vi "Main.vi"() -> ()   [LabVIEW 2025]
uses:
  TypeDef_AuxPlotValues.ctl
  TypeDef_AuxDataToDisplay.ctl
  TypeDef_Modes.ctl
  TypeDef_BBBJSON_commands.ctl
  TypeDef_Network.ctl
  <vilib>/Analysis/1siggen.llb/Ramp Pattern by Samples.vi
  <vilib>/Analysis/NI_AALBase.lvlib
panel:
  out "Gly Conc (ppb)":dbl
  out "NO2 Conc (ppb)":dbl
  out "Laptop loop time":dbl
  out "Laptop Time":timestamp
  out "Aux data to display":T1={"LED T"=0.0, "Sink T"=0.0, "TEC Current"=0.0, "TEC Voltage"=0.0, "Is LED T stable?"=FALSE, "Is TEC enabled?"=FALSE, "TEC Status"=enum."Error", "Cavity Flow"=0.0, "Cavity Flow Setpoint"=0.0, "Overflow"=0.0, "Overflow Setpoint"=0.0, "LED Current"=0.0, "Cavity Pressure"=0.0, "Cavity T"=0.0, "Box T"=0.0, "LED on/off"=FALSE, "ZA/He valve"=FALSE, "NO2 add valve"=FALSE}
  out "Spectrum type":u32
  out "Current file":string
  in  "Start saving":bool
  out "Message to BBB":string
  out "Auto signal to BBB?":bool
  out "Auto valves":bool[][](array[boolean])
  out "Auto flows":dbl[][](array[numeric])
  in  "Do it now":T2
  out "Substate":string
  out "Action times":cluster{dbl[], dbl[]} {"?" format="%.2f"; "?" format="%<%H:%M:%S>t"}
  out "Time left":dbl
  in  "Abort action":bool
  in  "Auto actions":bool[](array[boolean])
  in  "Reset?":T3
  out "Action Queue":string[](array[string])
  out "Current state":i32
  in  "Clear queue":bool
  out "Actions":string[](array[string])
  out "BBB time":timestamp
  in  "stop":bool
  in  "Tab Control":T4(tab)
  out "Chosen wavelength":dbl
  in  "Max minutes to plot":dbl=30.0
  in  "Pixel":i32=500
  out "Aux data":cluster{dbl[], dbl[]}(graph)
  in  "Value To Plot":T5
  out "Spectral data:":cluster{dbl[], dbl[]}(graph)
  in  "Spec plot":enum16{"Counts", "Ext", "Conc", "Auto"}(ring)=enum."Auto"
  out "Dark":cluster{"Wavelength":dbl[], "Ch1 Dark":dbl[]}(graph)
  out "R Alpha":cluster{"Wavelength":dbl[], "Array out":dbl[]}(graph)
  in  "LED temperature threshold (deg C)":dbl=30.0
  in  "LED safety override enabled?":bool=TRUE
  in  "Reset TEC":bool
  in  "Cooling enabled":bool=TRUE
  in  "User flows (vlpm)":dbl[](array[numeric])=[0.0, 0.0]
  in  "User valves":bool[](array[boolean])=[FALSE, FALSE, FALSE]
  in  "TEC set point":dbl=25.0
  in  "Config file name":path=path "C:/Users/ceslab/Documents/pyCESViewer/CES_Config.ini"
  # "Read out from BBB:"
  # "Auto states:"
  # "Channel flow"
  # "Overflow"
  # "ZA/He valve"
  # "NO2 valve"
  # "LED on/off"
  # "(Only works on TEC FW>5, I think?)"
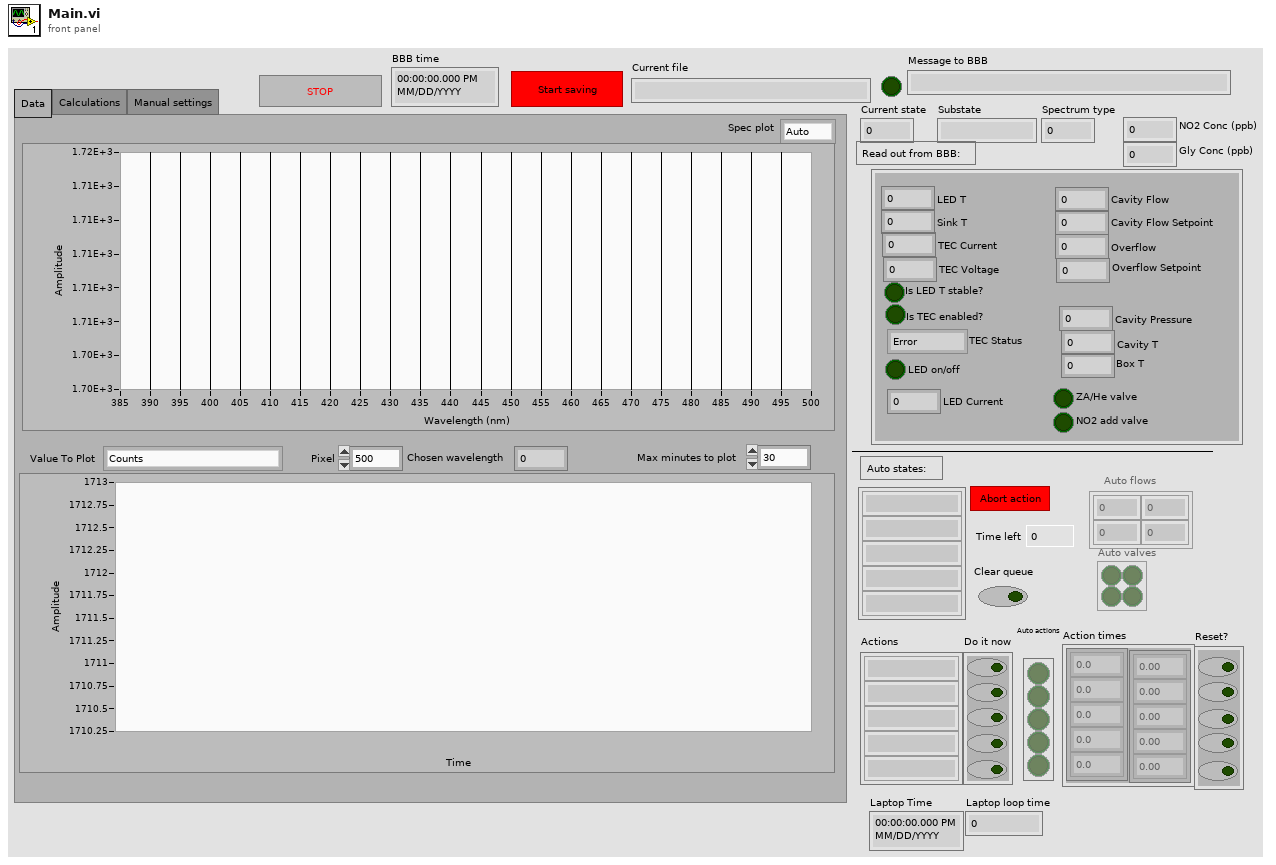
[diagram p1: front panel]
types:
  T1 = typedef "TypeDef_AuxDataToDisplay.ctl" = cluster{"LED T":dbl, "Sink T":dbl, "TEC Current":dbl, "TEC Voltage":dbl, "Is LED T stable?":bool, "Is TEC enabled?":bool, "TEC Status":enum16{"Initializing", "Idle", "Running", "Error", "Bootloader", "Device restarting"}, "Cavity Flow":dbl, "Cavity Flow Setpoint":dbl, "Overflow":dbl, "Overflow Setpoint":dbl, "LED Current":dbl, "Cavity Pressure":dbl, "Cavity T":dbl, "Box T":dbl, "LED on/off":bool, "ZA/He valve":bool, "NO2 add valve":bool}
  T2 = cluster{"Action 1":bool, "Action 2":bool, "Action 3":bool, "Action 4":bool, "Action 5":bool}
  T3 = cluster{"Reset 1":bool, "Reset 2":bool, "Reset 3":bool, "Reset 4":bool, "Reset 5":bool}
  T4 = enum32{"Data", "Calculations", "Manual settings"}
  T5 = typedef "TypeDef_AuxPlotValues.ctl" = enum16{"Counts", "LED T", "Sink T", "Target T", "TEC Current", "TEC Voltage", "Is LED T stable?", "Is TEC enabled?", "TEC Status", "MFC Cavity Flow", "MFC Cavity Flow Setpoint", "MFC Cavity Flow Temperature", "MFC Cavity Flow Pressure", "MFC Overflow", "MFC Overflow Setpoint", "MFC Overflow Temperature", "MFC Overflow Pressure", "LED current", "Cavity Pressure", "Cavity T", "Box T", "LED on/off", "ZA/He valve", "NO2 valve", "State number", "NO2 concentration", "Glyoxal concentration"}
  T6 = typedef "TypeDef_Modes.ctl" = enum16{"Initialize", "ReadFromBB", "Idle", "SendCMDtoBB", "Shutdown"}
  T7 = enum16{"Spectrometer", "Calculations", "BBB", "States", "Actions"}
  T8 = typedef "TypeDef_BBBJSON_commands.ctl" = cluster{"SetState":cluster{"StateNum":i32}, "SetSave":cluster{"Save":i16}, "SetTEC":cluster{"TargetT":dbl, "Reset":i32, "Enable":i32}, "SetMFC":cluster{"MFC0":dbl, "MFC1":dbl}, "SetGPIO":cluster{"SSR0":i16, "SSR1":i16, "LED":i16}}
  T9 = typedef "TypeDef_Network.ctl" = cluster{"port name":refnum<k16>, "server IP address":u32, "server port":u16, "client IP address":u32, "client port":u16, "max_bytes":i32, "timeout_us":i32}
  T10 = typedef "TypeDef_SpectrometerConfigData.ctl" = cluster{"pixels":i32, "start wavelength":dbl, "stop wavelength":dbl}
  T11 = typedef "TypeDef_DataIn.ctl" = cluster{"TEC data":cluster{"stat":i32, "Tstb":i32, "enab":i32, "objT":dbl, "snkT":dbl, "tarT":dbl, "tecI":dbl, "tecV":dbl}, "MFC data":cluster{"cavityFlow":cluster{"Unit":string, "temperature":dbl, "flow":dbl, "setpoint":dbl, "gas":string}, "overflow":cluster{"Unit":string, "temperature":dbl, "flow":dbl, "setpoint":dbl, "gas":string}}, "analog data":cluster{"Therm0":dbl, "Therm1":dbl, "Therm2":dbl, "Press":dbl, "LED_Curr":dbl, "Vin_Volt":dbl, "Spare":dbl}, "gpio data":cluster{"SSR0":i32, "SSR1":i32, "LED":i32}}
  T12 = typedef "TypeDef_AuxDataToPlot.ctl" = cluster{"LED T":dbl, "Sink T":dbl, "TEC Target T":dbl, "TEC Current":dbl, "TEC Voltage":dbl, "Is LED T stable?":dbl, "TEC Status":dbl, "Is TEC enabled?":dbl, "MFC Cavity Flow":dbl, "MFC Cavity Flow Setpoint":dbl, "MFC Cavity Flow Temperature":dbl, "MFC Cavity Flow Pressure":dbl, "MFC Overflow":dbl, "MFC Overflow Setpoint":dbl, "MFC Overflow Temperature":dbl, "MFC Overflow Pressure ":dbl, "LED Current":dbl, "Cavity Pressure":dbl, "Cavity T":dbl, "Box T":dbl, "LED on/off":dbl, "ZA/He valve":dbl, "NO2 add valve":dbl}
  T13 = cluster{"Ramp Pattern":dbl[], "Spectral Data":dbl[]}
  T14 = cluster{"Flows":dbl[][], "Valves":bool[][], "Flags":i32[]}
  T15 = cluster{"TargetT":dbl, "Reset":i32, "Enable":i32}
  T16 = cluster{"SetTEC":cluster{"TargetT":dbl, "Reset":i32, "Enable":i32}}
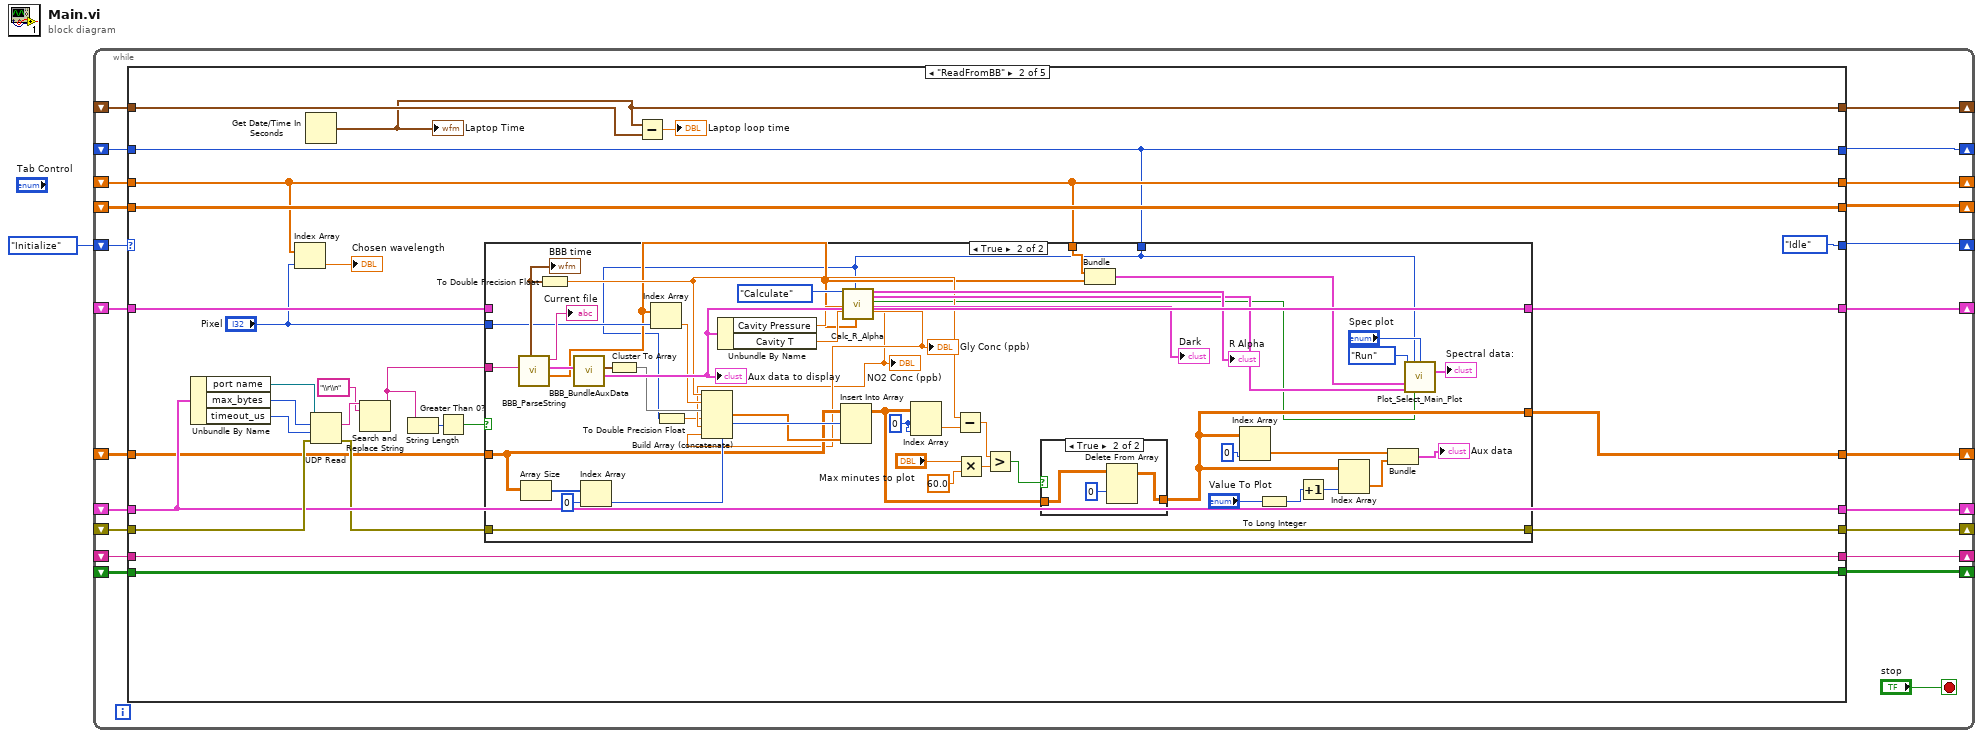
[diagram p0: block diagram]
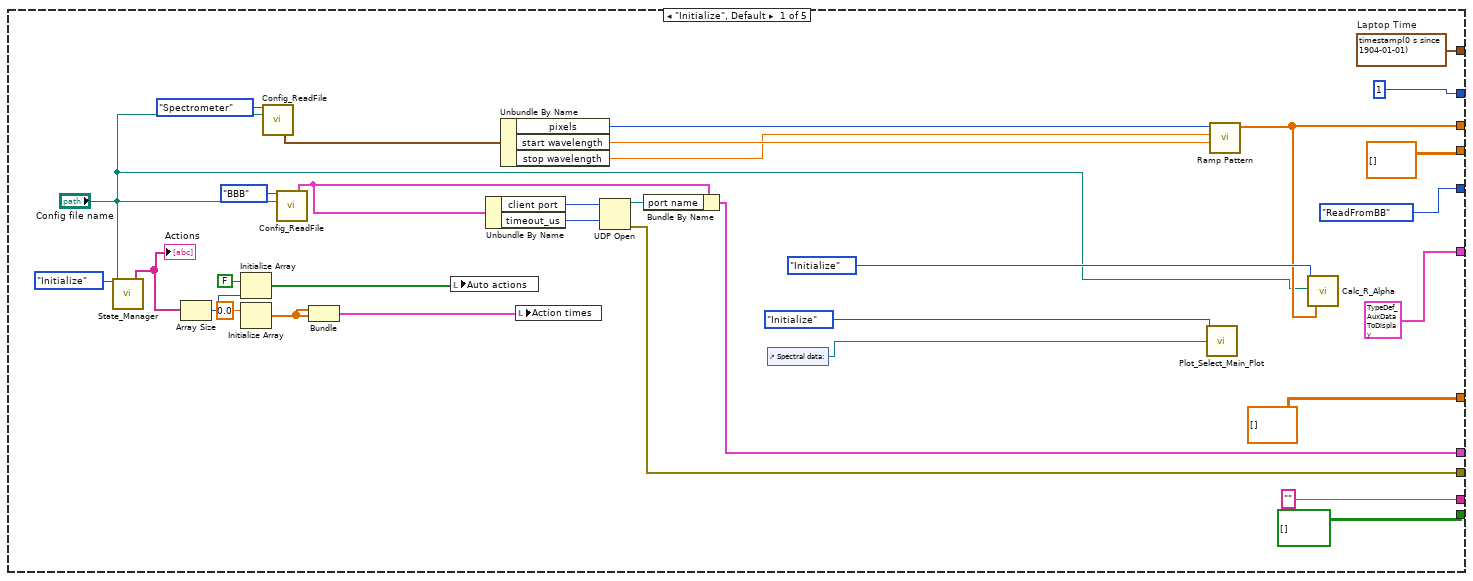
[diagram p2: hidden frame]
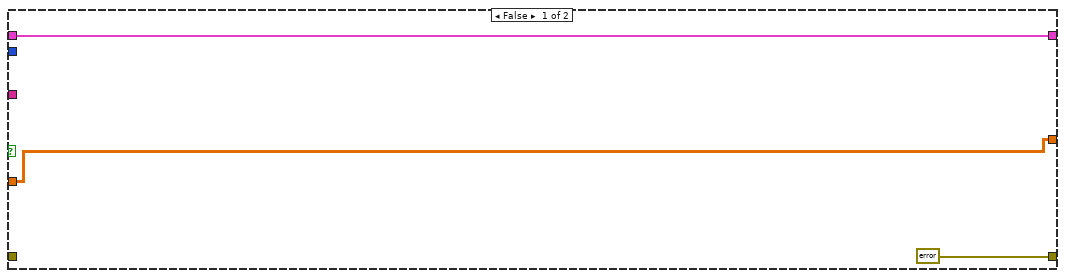
[diagram p3: hidden frame]
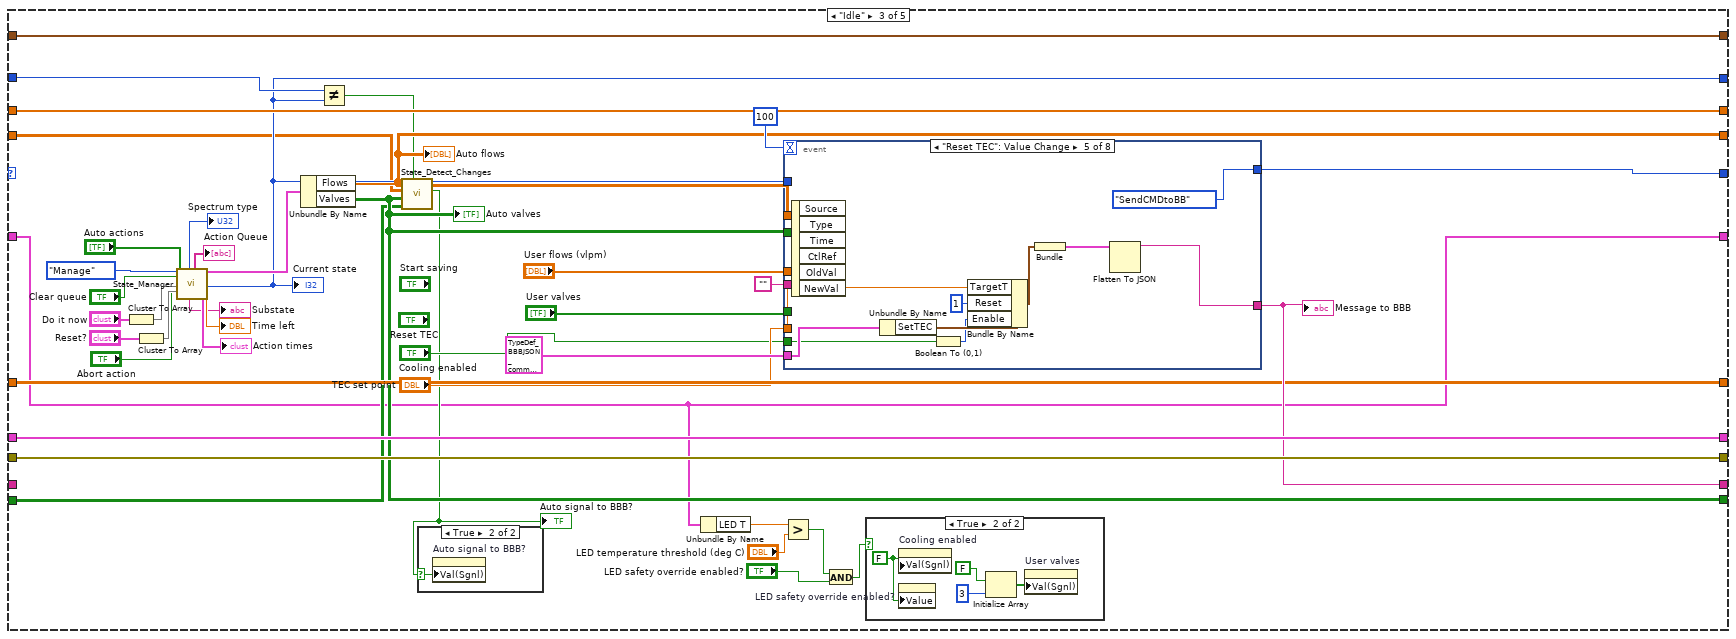
[diagram p5: hidden frame]
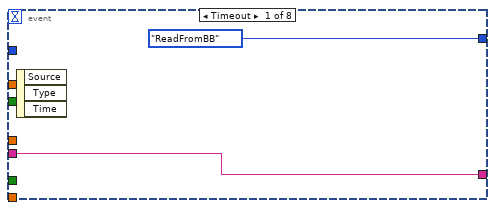
[diagram p8: hidden frame]
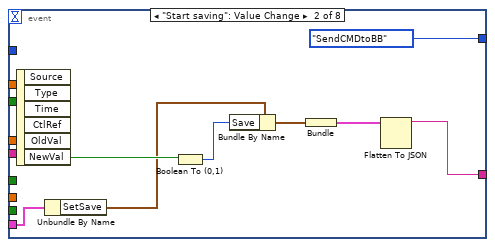
[diagram p9: hidden frame]
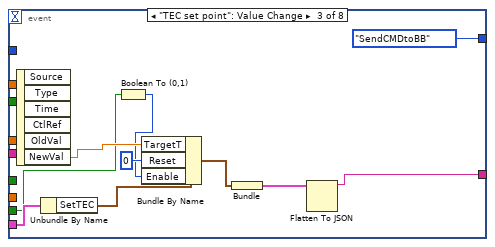
[diagram p10: hidden frame]
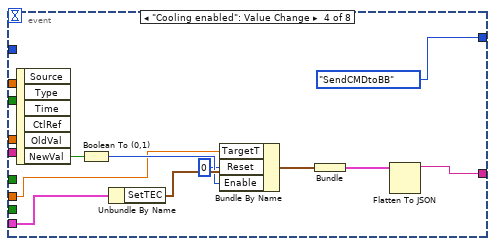
[diagram p11: hidden frame]
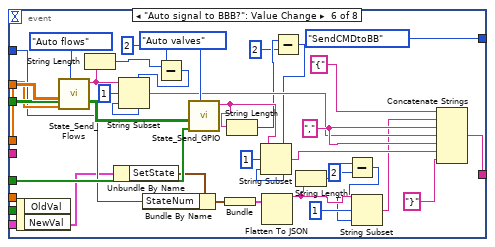
[diagram p12: hidden frame]
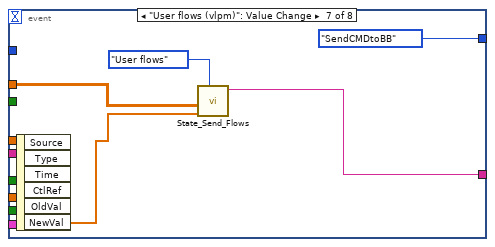
[diagram p13: hidden frame]
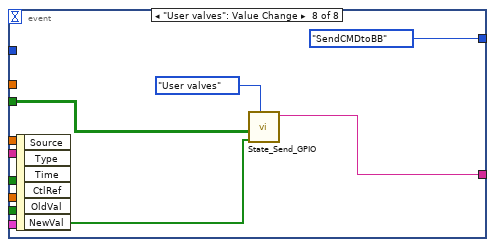
[diagram p14: hidden frame]
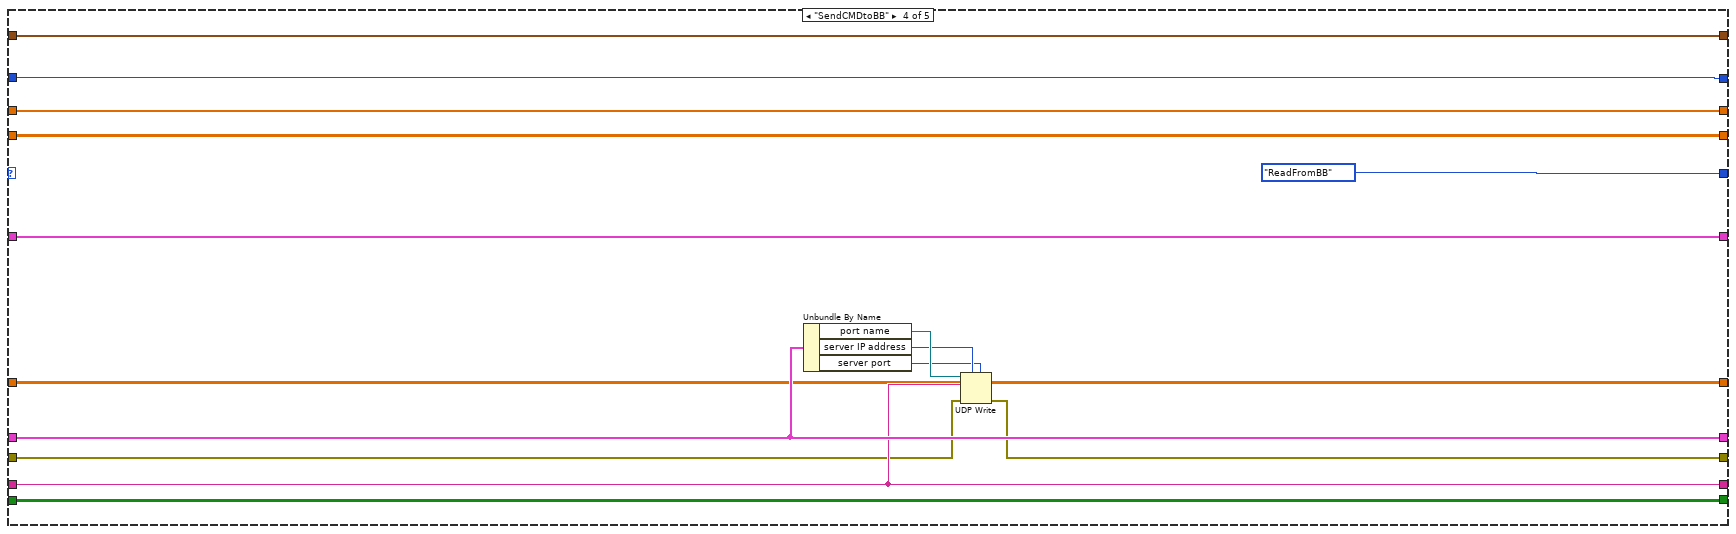
[diagram p15: hidden frame]
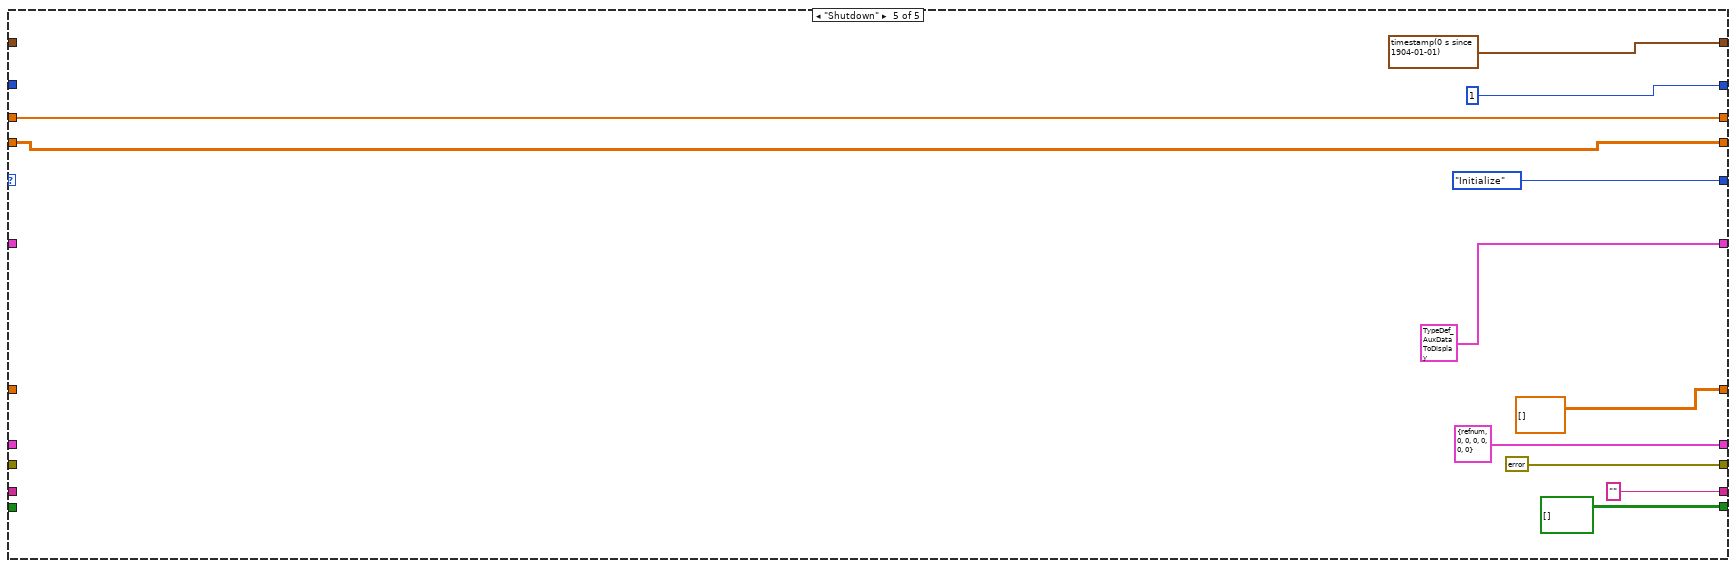
[diagram p16: hidden frame]
diagram:
  n1 = while {
    shift-right: [w21] -> _
    shift-left: TypeDef_Modes."Initialize" ("Enum") -> [w24]
    shift-right: [w4] -> _
    shift-left: _ -> [w22]
    shift-right: [w3] -> _
    shift-left: _ -> [w20]
    shift-right: [w5] -> _
    shift-left: _ -> [w19]
    shift-right: [w8] -> _
    shift-left: _ -> [w18]
    shift-right: [w7] -> _
    shift-left: _ -> [w17]
    shift-right: [w16] -> _
    shift-left: _ -> [w15]
    shift-right: [w2] -> _
    shift-left: _ -> [w14]
    shift-right: [w13] -> _
    shift-left: _ -> [w12]
    shift-right: [w6] -> _
    shift-left: _ -> [w11]
    shift-right: [w10] -> _
    shift-left: _ -> [w9]
    stop <- "stop" stop-if-true
    n2 = case shown="\"ReadFromBB\"" w24 {
      tunnel: [w44 w59 w181 w282 errorcluster {"status"=FALSE, "code"=0, "source"=""} ("error out")] -> w4
      tunnel: w22 -> [_ w84 w181 w281 _]
      tunnel: [TypeDef_Modes."ReadFromBB" ("Enum") TypeDef_Modes."Idle" ("Enum") w180 TypeDef_Modes."ReadFromBB" ("Enum") TypeDef_Modes."Initialize" ("Enum")] -> w21
      tunnel: ["" w83 w179 w284 ""] -> w3
      tunnel: w20 -> [_ w83 _ w284 _]
      tunnel: [w30 w81 w182 w285 T9 {"port name"=refnum, "server IP address"=0, "server port"=0, "client IP address"=0, "client port"=0, "max_bytes"=0, "timeout_us"=0} ("cluster")] -> w5
      tunnel: w19 -> [_ w81 w182 w285 _]
      tunnel: [dbl[][] [] w62 w177 w278 dbl[][] []] -> w8
      tunnel: w18 -> [_ w64 w177 w278 _]
      tunnel: [w42 w61 w164 w277 w292] -> w7
      tunnel: w17 -> [_ w61 w164 w277 w292]
      tunnel: [dbl[][] [] ("Flows") w80 w155 w276 w290] -> w16
      tunnel: w15 -> [_ w80 w152 w276 w290]
      tunnel: [bool[][] [] ("Valves") w79 w154 w275 bool[][] [] ("Valves")] -> w2
      tunnel: w14 -> [_ w79 w153 w275 _]
      tunnel: [1 ("Current state") w60 w160 w274 1 ("Current state")] -> w13
      tunnel: w12 -> [_ w60 w161 w274 _]
      tunnel: [T1 {"LED T"=0.0, "Sink T"=0.0, "TEC Current"=0.0, "TEC Voltage"=0.0, "Is LED T stable?"=FALSE, "Is TEC enabled?"=FALSE, "TEC Status"=enum."Initializing", "Cavity Flow"=0.0, "Cavity Flow Setpoint"=0.0, "Overflow"=0.0, "Overflow Setpoint"=0.0, "LED Current"=0.0, "Cavity Pressure"=0.0, "Cavity T"=0.0, "Box T"=0.0, "LED on/off"=FALSE, "ZA/He valve"=FALSE, "NO2 add valve"=FALSE} ("Aux data to display") w58 w147 w273 T1 {"LED T"=0.0, "Sink T"=0.0, "TEC Current"=0.0, "TEC Voltage"=0.0, "Is LED T stable?"=FALSE, "Is TEC enabled?"=FALSE, "TEC Status"=enum."Initializing", "Cavity Flow"=0.0, "Cavity Flow Setpoint"=0.0, "Overflow"=0.0, "Overflow Setpoint"=0.0, "LED Current"=0.0, "Cavity Pressure"=0.0, "Cavity T"=0.0, "Box T"=0.0, "LED on/off"=FALSE, "ZA/He valve"=FALSE, "NO2 add valve"=FALSE} ("Aux data to display")] -> w6
      tunnel: w11 -> [_ w71 w147 w273 _]
      tunnel: [w37 w69 w149 w272 timestamp(0 s since 1904-01-01) ("seconds since 1Jan1904")] -> w10
      tunnel: w9 -> [_ w70 w149 w272 _]
      frame "Initialize", Default {
        w37 = timestamp(0 s since 1904-01-01)  # Laptop Time
        n3 = call "State_Manager.vi"("Mode"=enum16{"Initialize", "Manage", "Close"}."Initialize", "Config file name"="Config file name") -> ("Action list"=w50:string[])  [unwired: 9 in, 8 out]
        "Actions" <- w50
        n4 = Array Size(array=w50) -> (size(s)=w51:i32)
        n5 = Initialize Array(FALSE, w51) -> (w53:bool[])
        n6 = Initialize Array(0.0) -> (w52:dbl[])  [unwired: 1 in]
        n7 = call "Config_ReadFile.vi"("Section"=T7."Spectrometer", "Config file name"="Config file name") -> ("Spectrometer config data"=w36:T10)  [unwired: 7 in, 6 out]
        n8 = call "Config_ReadFile.vi"("Section"=T7."BBB", "Config file name"="Config file name") -> ("BBB config data"=w32:T9)  [unwired: 7 in, 6 out]
        n9 = Bundle(w52, w52) -> (w54:cluster{dbl[], dbl[]})  [unwired: 1 in]
        n10 = local write "Auto actions"(w53) -> ()
        n11 = Unbundle By Name(w32) -> ("client port"=w29:u16, "timeout_us"=w28:i32)
        n12 = Unbundle By Name(w36) -> ("pixels"=w35:i32, "start wavelength"=w34:dbl, "stop wavelength"=w33:dbl)
        n13 = local write "Action times"(w54) -> ()
        n14 = UDP Open(9:w28, 11:w29) -> (port=w31:refnum<k16>, 0:w44:errorcluster)  [unwired: 3 in, 1 out]
        n15 = Bundle By Name(cluster=w32, "port name"=w31) -> (w30:T9)
        n16 = control-ref of="Spectral data:"() -> (w40:refnum<vi>)
        n17 = call "Plot_Select_Main_Plot.vi"("Mode"=enum16{"Initialize", "Run"}."Initialize", "Spectra"=w40) -> ()  [unwired: 13 in, 1 out]
        n18 = call-poly <vilib>:"Ramp Pattern.vi"("start"=w34, "end"=w33, "samples"=w35) -> ("Ramp Pattern"=w42:dbl[])  [unwired: 7 in, 1 out]
        n19 = call "Calc_R_Alpha.vi"("Mode"=enum16{"Initialize", "Calculate"}."Initialize", "Config file name"="Config file name", "Wavelength"=w42) -> ()  [unwired: 10 in, 7 out]
      }
      frame "ReadFromBB" {
        n20 = Unbundle By Name(w81) -> ("port name"=w77:refnum<k16>, "max_bytes"=w67:i32, "timeout_us"=w66:i32)
        n21 = Index Array(array=w61, index="Pixel") -> (element=→"Chosen wavelength":dbl)
        n22 = Get Date/Time In Seconds() -> (seconds since 1Jan1904=w69:timestamp)
        "Laptop Time" <- w69
        n23 = UDP Read(connection ID=w77, max size (548)=w67, timeout ms (25000)=w66, 8:w84) -> (data out=w78:string, error out=w73:errorcluster)  [unwired: 3 out]
        n24 = Search and Replace String(input string=w78, search string="\\r\\n") -> (result string=w72:string)  [unwired: 6 in, 3 out]
        n25 = String Length(string=w72) -> (length=w75:i32)
        n26 = Greater Than 0?(x=w75) -> (x > 0?=w74:bool)
        n27 = case shown="True" w74 {
          tunnel: w73 -> [_ w136]
          tunnel: [errorcluster {"status"=FALSE, "code"=0, "source"=""} ("error out") w136] -> w59
          tunnel: w72 -> [_ w134]
          tunnel: [w86 w133] -> w58
          tunnel: w71 -> [w86 _]
          tunnel: w64 -> [w85 w122]
          tunnel: "Pixel" -> [_ w126]
          tunnel: [w85 w109] -> w62
          tunnel: w61 -> [_ w94]
          tunnel: w60 -> [_ w89]
          frame False {
          }
          frame True {
            w111 = 0 ("index (row)")
            n28 = call "BBB_ParseString.vi"("Input String"=w134) -> ("Spectral Data"=w92:dbl[], "Data out"=w131:T11, "file name"=→"Current file":string, "BBB Timestamp"=w132:timestamp)  [unwired: 5 in]
            "BBB time" <- w132
            n29 = Array Size(array=w122) -> (size(s)=w129:i32[])
            n30 = To Double Precision Float(number=w132) -> (double precision float=w96:dbl)
            n31 = call "BBB_BundleAuxData.vi"("Data in"=w131) -> ("Aux data to display"=w133:T1, "Aux data to Plot"=w135:T12)  [unwired: 9 in]
            "Aux data to display" <- w133
            n32 = Index Array(array=w129, index=0) -> (element=w128:i32)
            n33 = Cluster To Array(cluster=w135) -> (array=w125:dbl[])
            n34 = Index Array(array=w92, index=w126) -> (element=w127:dbl)
            n35 = To Double Precision Float(number=w89) -> (double precision float=w88:dbl)
            n36 = Unbundle By Name(w133) -> ("Cavity Pressure"=w98:dbl, "Cavity T"=w97:dbl)
            n37 = call "Calc_R_Alpha.vi"("Mode"=enum16{"Initialize", "Calculate"}."Calculate", "Pressure in"=w98, "Temperature In"=w97, "State in"=w89, "Spectra"=w92) -> ("NO2 Conc (ppb)"=w90:dbl, "Rs"=→"R Alpha":cluster{"Wavelength":dbl[], "Array out":dbl[]}, "Exts"=w103:cluster{"Wavelength":dbl[], "Array out":dbl[]}, "First?"=w93:bool, "Darks"=→"Dark":cluster{"Wavelength":dbl[], "Ch1 Dark":dbl[]}, "Gly Conc (ppb)"=w91:dbl)  [unwired: 8 in, 1 out]
            "NO2 Conc (ppb)" <- w90
            "Gly Conc (ppb)" <- w91
            n38 = Build Array (concatenate)(w96, w127, w125, w88, w90, w91) -> (w124:dbl[])
            n39 = Insert Into Array(array=w122, index (row)=w128, new element=w124) -> (w112:dbl[][])  [unwired: 1 in]
            n40 = Index Array(array=w112, index (row)=w111, index (col)=w111) -> (element=w115:dbl)
            n41 = Subtract(x=w96, y=w115) -> (x-y=w95:dbl)
            n42 = Multiply(x="Max minutes to plot", y=60.0) -> (x*y=w108:dbl)
            n43 = Greater?(x=w95, y=w108) -> (0:w107:bool)
            n44 = case shown="True" w107 {
              tunnel: w112 -> [w137 w140]
              tunnel: [w137 w139] -> w109
              frame False {
              }
              frame True {
                n45 = Delete From Array(array=w140, index (row)=0) -> (array with subset deleted=w139:dbl[][])  [unwired: 2 in, 1 out]
              }
            }
            n46 = Bundle("Ramp Pattern"=w94, "Spectral Data"=w92) -> (w106:T13)  [unwired: 1 in]
            n47 = Index Array(array=w109, index (col)=0 ("index (row)")) -> (element=w121:dbl[])  [unwired: 1 in]
            n48 = To Long Integer(number="Value To Plot") -> (32bit integer=w117:i32)
            n49 = Increment(x=w117) -> (x+1=w116:i32)
            n50 = Index Array(array=w109, index (col)=w116) -> (element=w120:dbl[])  [unwired: 1 in]
            n51 = Bundle(w121, w120) -> (→"Aux data":cluster{dbl[], dbl[]})  [unwired: 1 in]
            n52 = call "Plot_Select_Main_Plot.vi"("Mode"=enum16{"Initialize", "Run"}."Run", "State in"=w89, "Spec plot"="Spec plot", "Counts"=w106, "Exts"=w103, "First?"=w93) -> ("Plots"=→"Spectral data:":cluster{"Wavelength":dbl[], "Extinction ":dbl[]})  [unwired: 9 in]
          }
        }
        n53 = Subtract(x=w69, y=w70) -> (x-y=→"Laptop loop time":dbl)
      }
      frame "Idle" {
        n54 = Cluster To Array(cluster="Do it now") -> (array=w165:bool[])
        n55 = Cluster To Array(cluster="Reset?") -> (array=w172:bool[])
        n56 = call "State_Manager.vi"("Mode"=enum16{"Initialize", "Manage", "Close"}."Manage", "Clear queue"="Clear queue", "Immediate actions"=w165, "Reset"=w172, "Auto actions"="Auto actions", "Abort action"="Abort action") -> ("Spectrum type"=→"Spectrum type":u32, "Substate"=→"Substate":string, "Action Queue"=→"Action Queue":string[], "Action times"=→"Action times":cluster{dbl[], dbl[]}, "Output cluster"=w163:T14, "Current state"=w160:i32, "Time left"=→"Time left":dbl)  [unwired: 5 in, 2 out]
        "Current state" <- w160
        n57 = Unbundle By Name(w163) -> ("Flows"=w155:dbl[][], "Valves"=w154:bool[][])
        "Auto flows" <- w155
        "Auto valves" <- w154
        n58 = Not Equal?(x=w161, y=w160) -> (x != y?=w151:bool)
        n59 = call "State_Detect_Changes.vi"("New state?"=w151, "Old valves"=w153, "New valves"=w154, "Old flows"=w152, "New flows"=w155) -> ("Values have changed"=w150:bool)  [unwired: 6 in]
        "Auto signal to BBB?" <- w150
        n60 = case shown="True" w150 {
          selector: w150 -> [_ w187]
          frame False {
          }
          frame True {
            n61 = property on="Auto signal to BBB?" class="Bool (strict)"("Val(Sgnl)"=w187) -> ()  [unwired: 2 in, 2 out]
          }
        }
        n62 = Unbundle By Name(w147) -> ("LED T"=w141:dbl)
        n63 = Greater?(x=w141, y="LED temperature threshold (deg C)") -> (0:w145:bool)
        n64 = event shown="[4] \"Reset TEC\": Value Change" {
          selector: _ -> [_ _ _ _ _ _ _ _]
          dyn-events: _ -> [_ _ _ _ _ _ _ _]
          timeout: 100 -> [_ _ _ _ _ _ _ _]
          tunnel: [TypeDef_Modes."ReadFromBB" ("Enum") TypeDef_Modes."SendCMDtoBB" ("Enum") TypeDef_Modes."SendCMDtoBB" ("Enum") TypeDef_Modes."SendCMDtoBB" ("Enum") TypeDef_Modes."SendCMDtoBB" ("Enum") TypeDef_Modes."SendCMDtoBB" ("Enum") TypeDef_Modes."SendCMDtoBB" ("Enum") TypeDef_Modes."SendCMDtoBB" ("Enum")] -> w180
          tunnel: [w188 w190 w201 w211 w222 w253 w263 w268] -> w179
          tunnel: w155 -> [_ _ _ _ _ w260 w264 _]
          tunnel: w154 -> [_ _ _ _ _ w259 _ w269]
          tunnel: "User flows (vlpm)" -> [_ _ _ _ _ w256 _ _]
          tunnel: "" -> [w188 _ _ _ _ _ _ _]
          tunnel: "User valves" -> [_ _ _ _ _ w255 _ _]
          tunnel: w160 -> [_ _ _ _ _ w250 _ _]
          tunnel: T8 {"SetState"={"StateNum"=0}, "SetSave"={"Save"=0}, "SetTEC"={"TargetT"=0.0, "Reset"=0, "Enable"=0}, "SetMFC"={"MFC0"=0.0, "MFC1"=0.0}, "SetGPIO"={"SSR0"=0, "SSR1"=0, "LED"=0}} ("BBBcommands") -> [_ w195 w206 w217 w227 w228 _ _]
          tunnel: "TEC set point" -> [_ _ _ w209 w221 _ _ _]
          tunnel: "Cooling enabled" -> [_ _ w199 _ w220 _ _ _]
          event Timeout {
            n65 = event-data() -> ()  [unwired: 1 in, 3 out]
          }
          event "Start saving": Value Change {
            n66 = event-data() -> ("NewVal"=w196:bool)  [unwired: 1 in, 5 out]
            n67 = Unbundle By Name(w195) -> ("SetSave"=w194:cluster{"Save":i16})
            n68 = Boolean To (0,1)(Boolean=w196) -> (0, 1=w193:i16)
            n69 = Bundle By Name(cluster=w194, "Save"=w193) -> (w192:cluster{"Save":i16})
            n70 = Bundle("SetSave"=w192) -> (w191:cluster{"SetSave":cluster{"Save":i16}})  [unwired: 1 in]
            n71 = Flatten To JSON(anything=w191) -> (JSON string=w190:string)  [unwired: 2 in, 1 out]
          }
          event "TEC set point": Value Change {
            n72 = event-data() -> ("NewVal"=w204:dbl)  [unwired: 1 in, 5 out]
            n73 = Unbundle By Name(w206) -> ("SetTEC"=w205:T15)
            n74 = Boolean To (0,1)(Boolean=w199) -> (0, 1=w198:i16)
            n75 = Bundle By Name(cluster=w205, "TargetT"=w204, "Reset"=0, "Enable"=w198) -> (w203:T15)
            n76 = Bundle("SetTEC"=w203) -> (w202:T16)  [unwired: 1 in]
            n77 = Flatten To JSON(anything=w202) -> (JSON string=w201:string)  [unwired: 2 in, 1 out]
          }
          event "Cooling enabled": Value Change {
            n78 = event-data() -> ("NewVal"=w215:bool)  [unwired: 1 in, 5 out]
            n79 = Boolean To (0,1)(Boolean=w215) -> (0, 1=w214:i16)
            n80 = Unbundle By Name(w217) -> ("SetTEC"=w216:T15)
            n81 = Bundle By Name(cluster=w216, "TargetT"=w209, "Reset"=0, "Enable"=w214) -> (w213:T15)
            n82 = Bundle("SetTEC"=w213) -> (w212:T16)  [unwired: 1 in]
            n83 = Flatten To JSON(anything=w212) -> (JSON string=w211:string)  [unwired: 2 in, 1 out]
          }
          event "Reset TEC": Value Change {
            n84 = event-data() -> ()  [unwired: 1 in, 6 out]
            n85 = Unbundle By Name(w227) -> ("SetTEC"=w226:T15)
            n86 = Boolean To (0,1)(Boolean=w220) -> (0, 1=w219:i16)
            n87 = Bundle By Name(cluster=w226, "TargetT"=w221, "Reset"=1, "Enable"=w219) -> (w224:T15)
            n88 = Bundle("SetTEC"=w224) -> (w223:T16)  [unwired: 1 in]
            n89 = Flatten To JSON(anything=w223) -> (JSON string=w222:string)  [unwired: 2 in, 1 out]
          }
          event "Auto signal to BBB?": Value Change {
            w247 = "," ("string")
            n90 = event-data() -> ()  [unwired: 1 in, 2 out]
            n91 = call "State_Send_Flows.vi"("Mode"=enum16{"User flows", "Auto flows"}."Auto flows", "User flows in"=w256, "Auto flows in"=w260) -> ("BBB command out"=w245:string)  [unwired: 8 in]
            n92 = String Length(string=w245) -> (length=w237:i32)
            n93 = Unbundle By Name(w228) -> ("SetState"=w252:cluster{"StateNum":i32})
            n94 = Bundle By Name(cluster=w252, "StateNum"=w250) -> (w251:cluster{"StateNum":i32})
            n95 = Subtract(x=w237, y=2) -> (x-y=w235:i32)
            n96 = String Subset(string=w245, offset (0)=1, length (rest)=w235) -> (substring=w244:string)
            n97 = call "State_Send_GPIO.vi"("Mode"=enum16{"User valves", "Auto valves"}."Auto valves", "User valves in"=w255, "Auto valves in"=w259) -> ("BBB command out"=w242:string)  [unwired: 8 in]
            n98 = Bundle("SetState"=w251) -> (w249:cluster{"SetState":cluster{"StateNum":i32}})  [unwired: 1 in]
            n99 = String Length(string=w242) -> (length=w234:i32)
            n100 = Flatten To JSON(anything=w249) -> (JSON string=w239:string)  [unwired: 2 in, 1 out]
            n101 = Subtract(x=w234, y=2) -> (x-y=w233:i32)
            n102 = String Subset(string=w242, offset (0)=1, length (rest)=w233) -> (substring=w241:string)
            n103 = String Length(string=w239) -> (length=w231:i32)
            n104 = Subtract(x=w231, y=2) -> (x-y=w229:i32)
            n105 = String Subset(string=w239, offset (0)=1, length (rest)=w229) -> (substring=w238:string)
            n106 = Concatenate Strings("{" ("string"), w238, w247, w244, w247, w241, "}" ("string")) -> (w253:string)
          }
          event "User flows (vlpm)": Value Change {
            n107 = event-data() -> ("NewVal"=w262:dbl[])  [unwired: 1 in, 5 out]
            n108 = call "State_Send_Flows.vi"("Mode"=enum16{"User flows", "Auto flows"}."User flows", "User flows in"=w262, "Auto flows in"=w264) -> ("BBB command out"=w263:string)  [unwired: 8 in]
          }
          event "User valves": Value Change {
            n109 = event-data() -> ("NewVal"=w267:bool[])  [unwired: 1 in, 5 out]
            n110 = call "State_Send_GPIO.vi"("Mode"=enum16{"User valves", "Auto valves"}."User valves", "User valves in"=w267, "Auto valves in"=w269) -> ("BBB command out"=w268:string)  [unwired: 8 in]
          }
        }
        "Message to BBB" <- w179
        n111 = And(x=w145, y="LED safety override enabled?") -> (x .and. y?=w143:bool)
        n112 = case shown="True" w143 {
          frame False {
          }
          frame True {
            w183 = FALSE ("Cooling enabled")
            n113 = property on="Cooling enabled" class="Bool (strict)"("Val(Sgnl)"=w183) -> ()  [unwired: 2 in, 2 out]
            n114 = property on="LED safety override enabled?" class="Bool (strict)"("Value"=w183) -> ()  [unwired: 2 in, 2 out]
            n115 = Initialize Array(FALSE, 3 ("dimension size")) -> (w184:bool[])
            n116 = property on="User valves" class="Arr (strict)"("Val(Sgnl)"=w184) -> ()  [unwired: 2 in, 2 out]
          }
        }
      }
      frame "SendCMDtoBB" {
        n117 = Unbundle By Name(w285) -> ("port name"=w283:refnum<k16>, "server IP address"=w280:u32, "server port"=w279:u16)
        n118 = UDP Write(address=w280, port or service name=w279, connection ID=w283, data in=w284, 8:w281) -> (error out=w282:errorcluster)  [unwired: 1 in, 1 out]
      }
      frame "Shutdown" {
      }
    }
  }
